vi "getNamesFromPath.vi"(4 "error in (no error)":errorcluster, 7 "tree path":string) -> (0 "error out":errorcluster, 2 "channel":string, 3 "group":string)   [LabVIEW 2020]
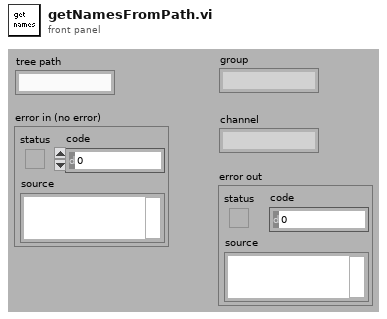
[diagram p1: front panel]
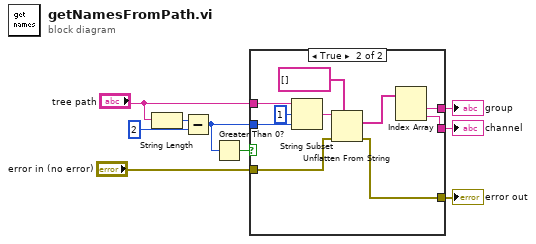
[diagram p0: block diagram]
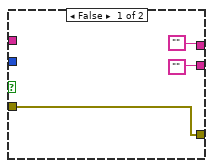
[diagram p2: hidden frame]
diagram:
  n1 = String Length(string="tree path") -> (length=w5:i32)
  n2 = Subtract(x=w5, y=2 ("offset (0)")) -> (x-y=w2:i32)
  n3 = Greater Than 0?(x=w2) -> (x > 0?=w1:bool)
  n4 = case shown="True" w1 {
    tunnel: [w10 w22] -> w9
    tunnel: "error in (no error)" -> [w10 w21]
    tunnel: "tree path" -> [_ w20]
    tunnel: w2 -> [_ w18]
    tunnel: ["" w16] -> w4
    tunnel: ["" w15] -> w3
    frame False {
    }
    frame True {
      n5 = String Subset(string=w20, offset (0)=1, length (rest)=w18) -> (substring=w19:string)
      n6 = Unflatten From String(type=string[] [], binary string=w19, error in (no error)=w21) -> (value=w14:string[], error out=w22:errorcluster)  [unwired: 2 in, 1 out]
      n7 = Index Array(array=w14) -> (element #1=w15:string, element #2=w16:string)  [unwired: 2 in]
    }
  }
  "error out" <- w9
  "channel" <- w4
  "group" <- w3
